vi "Update Picture Drag.vi"(8 "error in (no error)":errorcluster, 10 "picture mouse coordinate":cluster{"x":i32, "y":i32}, 11 "dialog info in":T1={"steering frame ref"=refnum, "active wheel indexes"=[], "FP Refs"={"VI Refnum"=refnum, "Menu Ref"=refnum, "Sub Panel"=refnum, "picture"=refnum, "Steering Type"=refnum, "zoom in"=refnum, "zoom out"=refnum, "zoom extents"=refnum, "Wheels"=refnum, "Add Wheel"=refnum, "Remove Wheel"=refnum, "Copy Wheel"=refnum, "Angle Units"=refnum}, "subpanel info"={"subpanel VI refs"=[], "subpanel types"=[], "main to subpanel command events"=[]}, "picture dragging state"={"dragging"=FALSE, "wheel index"=-1, "dragging mode"=enum."translate", "wheel start position"={"x"=0.0, "y"=0.0, "theta"=0.0}, "relative mouse position"={"x"=0.0, "y"=0.0}, "relative mouse init angle (rad)"=0.0}, "picture size (pixels)"={"Width"=500, "Height"=500}, "picture grid"=bytes[0], "click zones group"={"click zones array"=[], "num click zones"=0}, "draw options"={"draw wheel states?"=FALSE, "highlight wheel index"=-1, "pixels per unit"=10.0, "draw forward velocity?"=FALSE, "velocity scale"=1.0}}) -> (0 "error out":errorcluster, 3 "dialog info out":T1={"steering frame ref"=refnum, "active wheel indexes"=[], "FP Refs"={"VI Refnum"=refnum, "Menu Ref"=refnum, "Sub Panel"=refnum, "picture"=refnum, "Steering Type"=refnum, "zoom in"=refnum, "zoom out"=refnum, "zoom extents"=refnum, "Wheels"=refnum, "Add Wheel"=refnum, "Remove Wheel"=refnum, "Copy Wheel"=refnum, "Angle Units"=refnum}, "subpanel info"={"subpanel VI refs"=[], "subpanel types"=[], "main to subpanel command events"=[]}, "picture dragging state"={"dragging"=FALSE, "wheel index"=-1, "dragging mode"=enum."translate", "wheel start position"={"x"=0.0, "y"=0.0, "theta"=0.0}, "relative mouse position"={"x"=0.0, "y"=0.0}, "relative mouse init angle (rad)"=0.0}, "picture size (pixels)"={"Width"=500, "Height"=500}, "picture grid"=bytes[0], "click zones group"={"click zones array"=[], "num click zones"=0}, "draw options"={"draw wheel states?"=FALSE, "highlight wheel index"=-1, "pixels per unit"=10.0, "draw forward velocity?"=FALSE, "velocity scale"=1.0}})   [LabVIEW 2017, in "NI_Robotics_Configure Steering Frame.lvlib"]
uses:
  <vilib>/robotics/Dialog/Configure Steering Frame/NI_Robotics_Configure Steering Frame.lvlib
  <vilib>/robotics/Dialog/Configure Steering Frame/Dialog Info.ctl
  <vilib>/robotics/Steering/Steering Frame/NI_Robotics_Steering Frame.lvclass
  <vilib>/robotics/Dialog/Configure Steering Frame/FP Refs.ctl
  <vilib>/robotics/Dialog/Configure Steering Frame/Subpanel Info.ctl
  <vilib>/robotics/Dialog/Configure Steering Frame/Main to Subpanel Command Event.ctl
  <vilib>/robotics/Dialog/Configure Steering Frame/Main to Subpanel Command.ctl
  <vilib>/robotics/Dialog/Configure Steering Frame/Dragging State.ctl
  <vilib>/robotics/Dialog/Configure Steering Frame/Dragging Mode.ctl
  <vilib>/Utility/miscctls.llb/LVBoundsTypeDef.ctl
  <vilib>/robotics/Dialog/Configure Steering Frame/Click Zone.ctl
  <vilib>/robotics/Utilities/Visualization/Steering Visualization/Steering Picture/Draw Steering Frame Options.ctl
  <vilib>/robotics/Utilities/Visualization/Steering Visualization/Steering Picture/Picture Info.ctl
  <vilib>/robotics/Steering/Steering Frame/NI_Robotics_Steering Frame.lvclass/NI_Robotics_Steering Frame.ctl
  <vilib>/robotics/Steering/Wheel/NI_Robotics_Wheel.lvclass/NI_Robotics_Wheel.ctl
  <vilib>/robotics/Steering/Differential Steering Frame/NI_Robotics_Differential Steering Frame.lvclass/NI_Robotics_Differential Steering Frame.ctl
  <vilib>/robotics/Steering/Ackermann Steering Frame/NI_Robotics_Ackermann Steering Frame.lvclass/NI_Robotics_Ackermann Steering Frame.ctl
  <vilib>/robotics/Steering/Mecanum Steering Frame/NI_Robotics_Mecanum Steering Frame.lvclass/NI_Robotics_Mecanum Steering Frame.ctl
  <vilib>/Analysis/coordinate.llb/Angle Rotation (scalar).vi
  <vilib>/robotics/Dialog/Configure Steering Frame/Translate Wheel_Differential.vi
  <vilib>/robotics/Dialog/Configure Steering Frame/Translate Wheel_Ackermann.vi
  <vilib>/robotics/Dialog/Configure Steering Frame/Translate Wheel_Mecanum.vi
  <vilib>/Analysis/coordinate.llb/Wrap Angle (scalar).vi
  <vilib>/robotics/Steering/Differential Steering Frame/Set Wheel Separation.vi
  <vilib>/robotics/Steering/Ackermann Steering Frame/Get Wheel Separations.vi
  <vilib>/robotics/Steering/Ackermann Steering Frame/Set Wheel Separations.vi
  <vilib>/robotics/Steering/Mecanum Steering Frame/Set Wheel Separations.vi
  <vilib>/robotics/Steering/Differential Steering Frame/Wheel Separation to Frame Positions.vi
  <vilib>/robotics/Steering/Steering Frame/Reposition Wheels.vi
  <vilib>/robotics/Steering/Ackermann Steering Frame/Wheel Separation to Frame Positions.vi
  <vilib>/robotics/Steering/Mecanum Steering Frame/Wheel Separation to Frame Positions.vi
  <vilib>/robotics/Steering/Wheel/Update Steering to Wheel Frame Transform.vi
  <vilib>/Analysis/coordinate.llb/Wrap Angle.vi
  <vilib>/robotics/Steering/Differential Steering Frame/NI_Robotics_Differential Steering Frame.lvclass
  c:/Program Files (x86)/National Instruments/LabVIEW 2017/vi.lib/robotics/Steering/Steering Frame/NI_Robotics_Steering Frame.lvclass
  <vilib>/robotics/Steering/Ackermann Steering Frame/NI_Robotics_Ackermann Steering Frame.lvclass
  <vilib>/robotics/Steering/Mecanum Steering Frame/NI_Robotics_Mecanum Steering Frame.lvclass
  <vilib>/robotics/Steering/Steering Frame/Reposition Single Wheel on Steering Frame.vi
  <vilib>/robotics/Utilities/Visualization/Steering Visualization/Steering Picture/NI_Robotics_Steering Picture.lvlib
  <vilib>/Analysis/NI_AAL_Angle.lvlib
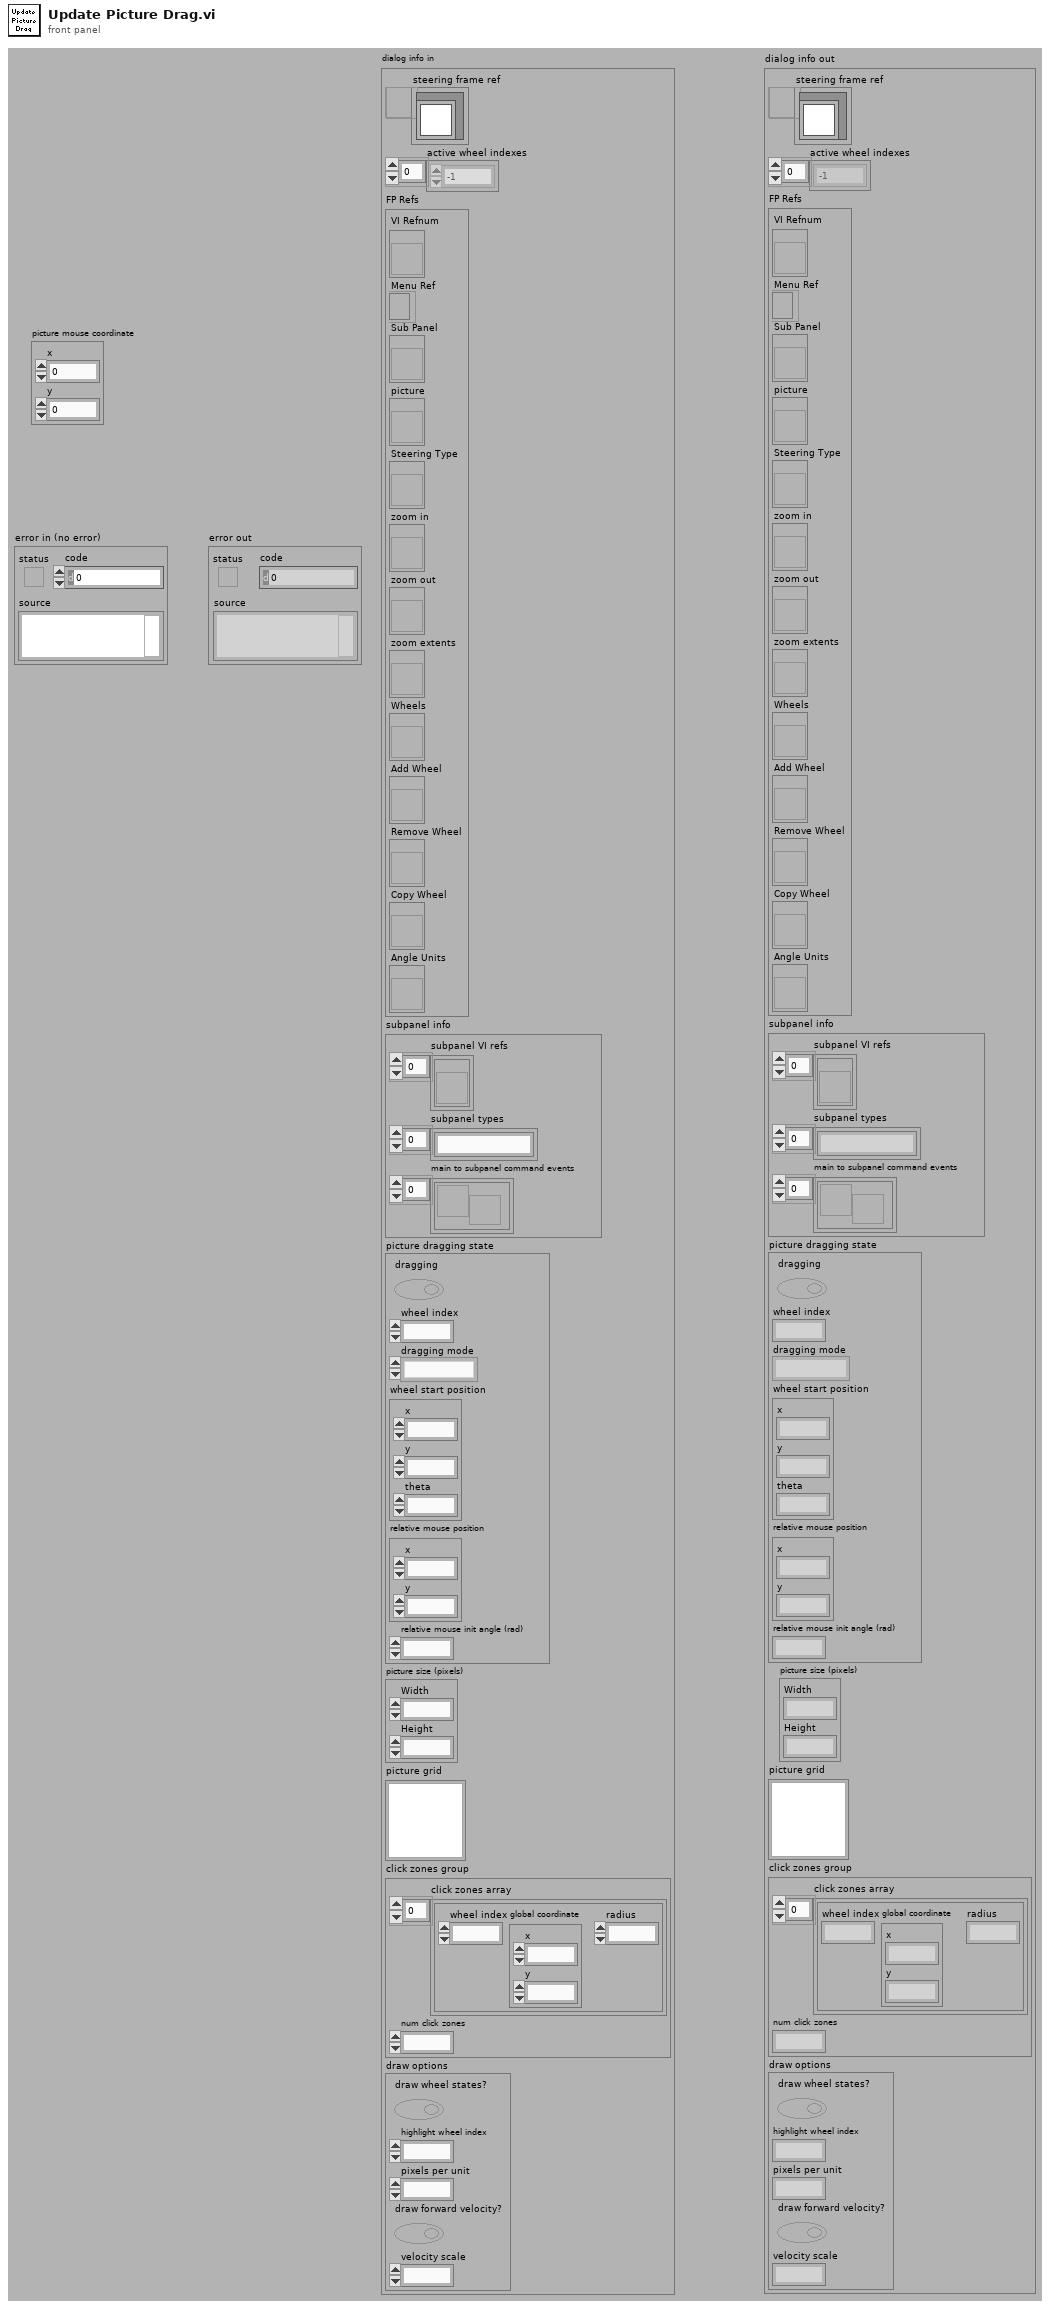
[diagram p1: front panel]
types:
  T1 = typedef "NI_Robotics_Configure Steering Frame.lvlib/Dialog Info.ctl" = cluster{"steering frame ref":refnum<data-value>, "active wheel indexes":i32[], "FP Refs":T2, "subpanel info":T3, "picture dragging state":T5, "picture size (pixels)":T7, "picture grid":picture, "click zones group":cluster{"click zones array":T8[], "num click zones":i32}, "draw options":T9}
  T2 = typedef "NI_Robotics_Configure Steering Frame.lvlib/FP Refs.ctl" = cluster{"VI Refnum":refnum<vi>, "Menu Ref":refnum<k9>, "Sub Panel":refnum<vi>, "picture":refnum<vi>, "Steering Type":refnum<vi>, "zoom in":refnum<vi>, "zoom out":refnum<vi>, "zoom extents":refnum<vi>, "Wheels":refnum<vi>, "Add Wheel":refnum<vi>, "Remove Wheel":refnum<vi>, "Copy Wheel":refnum<vi>, "Angle Units":refnum<vi>}
  T3 = typedef "NI_Robotics_Configure Steering Frame.lvlib/Subpanel Info.ctl" = cluster{"subpanel VI refs":refnum<vi>[], "subpanel types":string[], "main to subpanel command events":T4[]}
  T4 = typedef "NI_Robotics_Configure Steering Frame.lvlib/Main to Subpanel Command Event.ctl" = refnum<user-event>
  T5 = typedef "NI_Robotics_Configure Steering Frame.lvlib/Dragging State.ctl" = cluster{"dragging":bool, "wheel index":i32, "dragging mode":T6, "wheel start position":cluster{"x":dbl, "y":dbl, "theta":dbl}, "relative mouse position":cluster{"x":dbl, "y":dbl}, "relative mouse init angle (rad)":dbl}
  T6 = typedef "NI_Robotics_Configure Steering Frame.lvlib/Dragging Mode.ctl" = enum16{"translate", "rotate"}
  T7 = typedef "LVBoundsTypeDef.ctl" = cluster{"Width":u32, "Height":u32}
  T8 = typedef "NI_Robotics_Configure Steering Frame.lvlib/Click Zone.ctl" = cluster{"wheel index":i32, "global coordinate":cluster{"x":dbl, "y":dbl}, "radius":dbl}
  T9 = typedef "NI_Robotics_Steering Picture.lvlib/Draw Steering Frame Options.ctl" = cluster{"draw wheel states?":bool, "highlight wheel index":i32, "pixels per unit":dbl, "draw forward velocity?":bool, "velocity scale":dbl}
  T10 = typedef "NI_Robotics_Steering Picture.lvlib/Picture Info.ctl" = cluster{"picture size":T7, "pixels per unit":dbl}
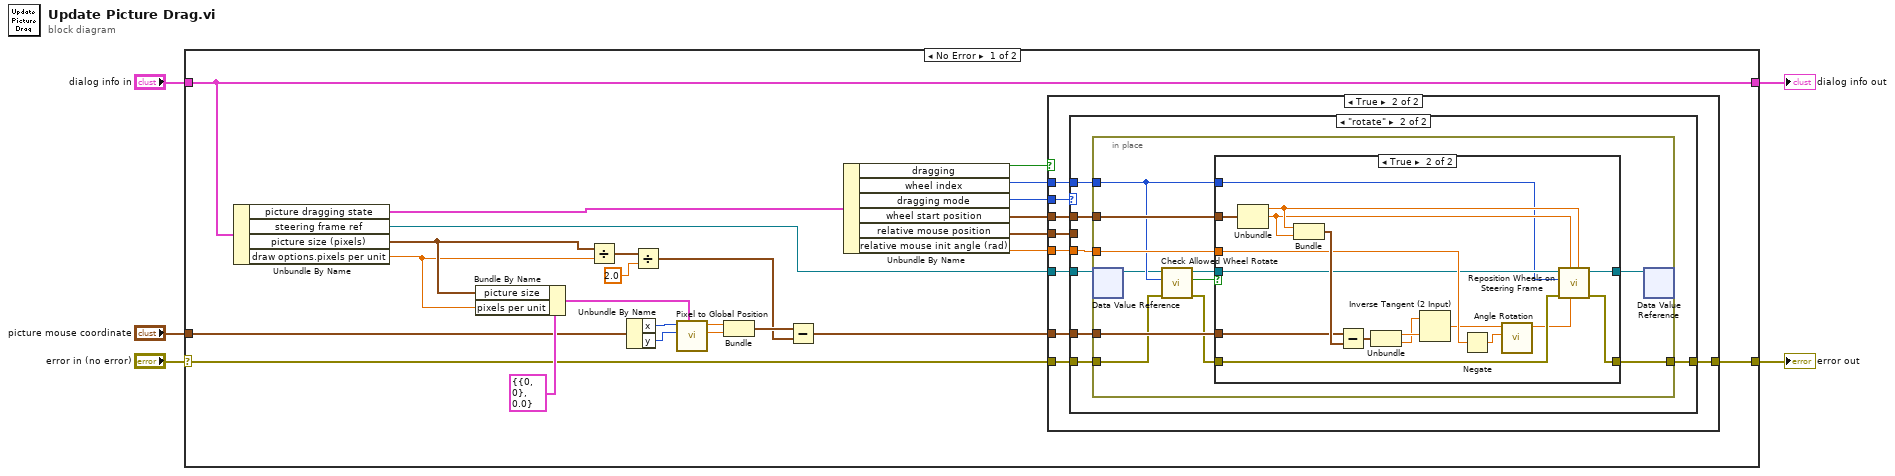
[diagram p0: block diagram]
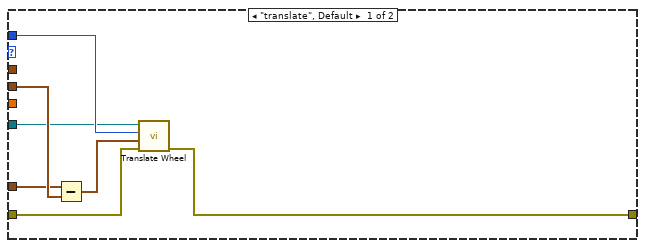
[diagram p3: hidden frame]
diagram:
  n1 = case shown="No Error" "error in (no error)" {
    selector: "error in (no error)" -> [w10 w86]
    tunnel: "dialog info in" -> [w8 w85]
    tunnel: [w9 w86] -> w3
    tunnel: [w8 w85] -> w2
    tunnel: "picture mouse coordinate" -> [w20 _]
    frame No Error {
      n2 = Unbundle By Name(w8) -> ("picture dragging state"=w11:T5, "steering frame ref"=w7:refnum<data-value>, "picture size (pixels)"=w27:T7, "draw options.pixels per unit"=w6:dbl)
      n3 = Bundle By Name(cluster=T10 {"picture size"={"Width"=0, "Height"=0}, "pixels per unit"=0.0} ("picture info"), "picture size"=w27, "pixels per unit"=w6) -> (w21:T10)
      n4 = Divide(x=w27, y=w6) -> (x/y=w30:cluster{"Width":dbl, "Height":dbl})
      n5 = Unbundle By Name(w20) -> ("x"=w23:i32, "y"=w22:i32)
      n6 = Divide(x=w30, y=2.0) -> (x/y=w19:cluster{"Width":dbl, "Height":dbl})
      n7 = call <vilib>:"Pixel to Global Position.vi"("picture info"=w21, "pixel y"=w22, "pixel x"=w23) -> ("global y"=w25:dbl, "global x"=w24:dbl)  [unwired: 7 in]
      n8 = Bundle("global x"=w24, "global y"=w25) -> (w26:cluster{"global x":dbl, "global y":dbl})  [unwired: 1 in]
      n9 = Subtract(x=w26, y=w19) -> (x-y=w12:cluster{dbl, dbl})
      n10 = Unbundle By Name(w11) -> ("dragging"=w18:bool, "wheel index"=w17:i32, "dragging mode"=w16:T6, "wheel start position"=w15:cluster{"x":dbl, "y":dbl, "theta":dbl}, "relative mouse position"=w14:cluster{"x":dbl, "y":dbl}, "relative mouse init angle (rad)"=w13:dbl)
      n11 = case shown="True" w18 {
        tunnel: w17 -> [_ w36]
        tunnel: w16 -> [_ w35]
        tunnel: w14 -> [_ w38]
        tunnel: w12 -> [_ w39]
        tunnel: [w31 w37] -> w9
        tunnel: w10 -> [w31 w40]
        tunnel: w13 -> [_ w34]
        tunnel: w15 -> [_ w33]
        tunnel: w7 -> [_ w32]
        frame False {
        }
        frame True {
          n12 = case shown="\"rotate\"" w35 {
            tunnel: w40 -> [w43 w49]
            tunnel: w39 -> [w46 w52]
            tunnel: w38 -> [w47 _]
            tunnel: [w42 w53] -> w37
            tunnel: w36 -> [w45 w50]
            tunnel: w34 -> [_ w51]
            tunnel: w33 -> [_ w54]
            tunnel: w32 -> [w41 w48]
            frame "translate", Default {
              n13 = Subtract(x=w46, y=w47) -> (x-y=w44:cluster{dbl, dbl})
              n14 = call <vilib>:"Translate Wheel.vi"("error in (no error)"=w43, "new position"=w44, "wheel index"=w45, "steering frame ref in"=w41) -> ("error out"=w42:errorcluster)  [unwired: 6 in, 1 out]
            }
            frame "rotate" {
              n15 = in-place {
                in-place-border: w54 -> [w65]
                in-place-border: [w64] -> w53
                in-place-border: w52 -> [w63]
                in-place-border: w51 -> [w62]
                in-place-border: w50 -> [w60]
                in-place-border: w49 -> [w59]
                n16 = in-place-dvr #1(w48) -> (w56:refnum<class "NI_Robotics_Steering Frame.lvclass">)  [unwired: 1 out]
                n17 = call <vilib>:"Check Allowed Wheel Rotate.vi"("error in (no error)"=w59, "wheel index"=w60, "steering frame in"=w56) -> ("error out"=w58:errorcluster, "rotate allowed?"=w57:bool, "steering frame out"=w61:refnum<class "NI_Robotics_Steering Frame.lvclass">)  [unwired: 6 in]
                n18 = case shown="True" w57 {
                  tunnel: [w67 w84] -> w55
                  tunnel: w65 -> [_ w83]
                  tunnel: [w66 w78] -> w64
                  tunnel: w63 -> [_ w75]
                  tunnel: w62 -> [_ w74]
                  tunnel: w61 -> [w67 w73]
                  tunnel: w60 -> [_ w72]
                  tunnel: w58 -> [w66 w71]
                  frame False {
                  }
                  frame True {
                    n19 = Unbundle(w83) -> ("x"=w77:dbl, "y"=w76:dbl)  [unwired: 1 out]
                    n20 = Bundle("x"=w77, "y"=w76) -> (w82:cluster{"x":dbl, "y":dbl})  [unwired: 1 in]
                    n21 = Subtract(x=w75, y=w82) -> (x-y=w81:cluster{dbl, dbl})
                    n22 = Unbundle(w81) -> (w80:dbl, w79:dbl)
                    n23 = Inverse Tangent (2 Input)(1:w80, 2:w79) -> (0:w70:dbl)
                    n24 = Negate(x=w74) -> (-x=w68:dbl)
                    n25 = call-poly <vilib>:"Angle Rotation.vi"("counterclockwise rotation"=w68, "angle"=w70) -> ("rotated angle"=w69:dbl)  [unwired: 8 in, 1 out]
                    n26 = call-poly <vilib>:"Reposition Wheels on Steering Frame.vi"("x position"=w77, "frame angle (rad)"=w69, "y position"=w76, "error in (no error)"=w71, "wheel index"=w72, "steering frame in"=w73) -> ("error out"=w78:errorcluster, "steering frame out"=w84:refnum<class "NI_Robotics_Steering Frame.lvclass">)  [unwired: 3 in, 1 out]
                  }
                }
                n27 = in-place-dvr #1(w55) -> ()  [unwired: 2 out]
              }
            }
          }
        }
      }
    }
    frame Error {
    }
  }
  "dialog info out" <- w2
  "error out" <- w3
